vi "Init Data.vi"(10 "Data":T1) -> (3 "Msg out":refnum<class "Msg.lvclass">)   [LabVIEW 2020, in "TcpClientHello.lvlib" / "Msg.lvclass"]
uses:
  Msg.lvclass
  Msg.lvclass/Msg.ctl
  Data.ctl
  TcpClientHello.lvlib
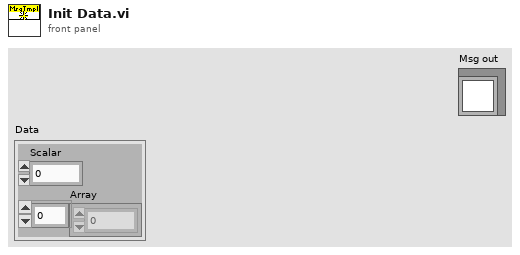
[diagram p1: front panel]
types:
  T1 = typedef "TcpClientHello.lvlib/Data.ctl" = cluster{"Scalar":dbl, "Array":dbl[]}
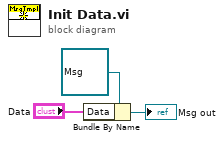
[diagram p0: block diagram]
diagram:
  n1 = Bundle By Name(cluster=refnum<class "Msg.lvclass"> refnum ("Msg out"), "Data"="Data") -> (→"Msg out":refnum<class "Msg.lvclass">)
